vi "AllThingsColors.vi"(8 "Choice":string) -> (3 "Possible Colors":string[](array[string]))   [LabVIEW 2022 SP3]
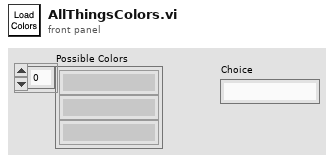
[diagram p1: front panel]
types:
  T1 = enum16{"big-endian, network order", "native, host order", "little-endian"}
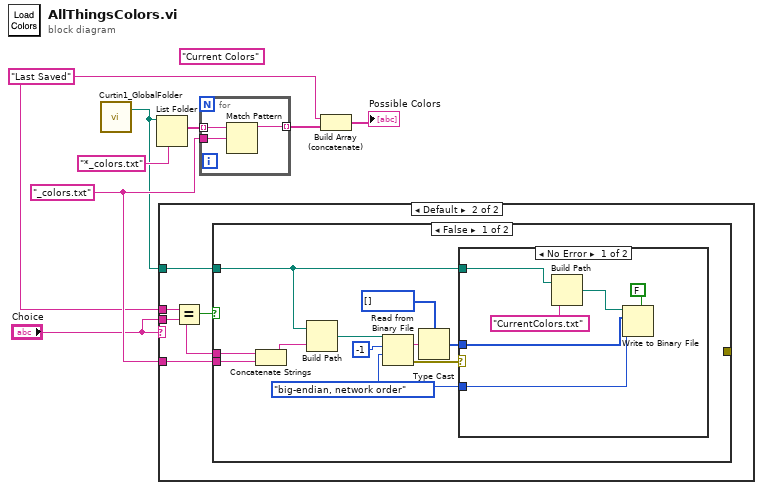
[diagram p0: block diagram]
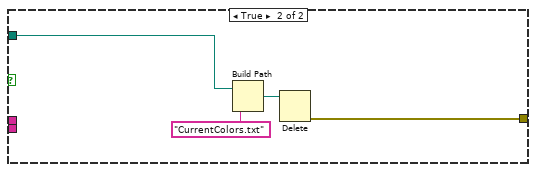
[diagram p4: hidden frame]
diagram:
  (unwired) "Current Colors" ("string")
  w4 = "_colors.txt" ("pattern")
  w3 = "Last Saved" ("string")
  n1 = call "Curtin1_GlobalFolder.vi"() -> ("LabVIEW Data Path"=w1:path)  [unwired: 1 in, 1 out]
  n2 = List Folder(path=w1, pattern="*_colors.txt") -> (filenames=w7:string[])  [unwired: 2 in, 3 out]
  n3 = case shown="Default" "Choice" {
    tunnel: w4 -> [_ w13]
    tunnel: "Choice" -> [_ w10]
    tunnel: w3 -> [_ w12]
    tunnel: w1 -> [_ w9]
    frame "" {
    }
    frame Default {
      n4 = Equal?(x=w12, y=w10) -> (x = y?=w11:bool)
      n5 = case shown="False" w11 {
        tunnel: w13 -> [w24 _]
        tunnel: w10 -> [w15 _]
        tunnel: [_ w32] -> _
        tunnel: w9 -> [w14 w31]
        frame False {
          w16 = T1."big-endian, network order" ("byte order (0:big-endian, network order)")
          n6 = Concatenate Strings(w15, w24) -> (w23:string)
          n7 = Build Path(base path=w14, name or relative path=w23) -> (appended path=w20:path)
          n8 = Read from Binary File(9:w16, 10:-1 ("count (1)"), 11:w20) -> (0:w19:errorcluster, 2:w21:string)  [unwired: 3 in, 2 out]
          n9 = Type Cast(type=u32[] [] ("Color"), x=w21) -> (*(type *) &x=w17:u32[])
          n10 = case shown="No Error" w19 {
            tunnel: w17 -> [w27 _]
            tunnel: w16 -> [w26 _]
            tunnel: w14 -> [w25 _]
            frame No Error {
              n11 = Build Path(base path=w25, name or relative path="CurrentColors.txt") -> (appended path=w28:path)
              n12 = Write to Binary File(file (use dialog)=w28, data=w27, 5:FALSE ("prepend array or string size? (T)"), 9:w26) -> ()  [unwired: 2 in, 3 out]
            }
            frame Error {
            }
          }
        }
        frame True {
          n13 = Build Path(base path=w31, name or relative path="CurrentColors.txt") -> (appended path=w33:path)
          n14 = Delete(path (use dialog)=w33) -> (error out=w32:errorcluster)  [unwired: 4 in, 2 out]
        }
      }
    }
  }
  n15 = for {
    tunnel: w7 -> [w37] mode=indexing
    tunnel: w4 -> [w36]
    tunnel: [w35] -> w8 mode=indexing
    n16 = Match Pattern(string=w37, regular expression=w36) -> (before substring=w35:string)  [unwired: 1 in, 3 out]
  }
  n17 = Build Array (concatenate)(w3, w8) -> (→"Possible Colors":string[])
